vi "Calculate INL.vi"(8 "Error In":errorcluster, 10 "V Zero":dbl, 11 "ADC in":refnum<class "ADC.lvclass">) -> (0 "Error Out":errorcluster, 2 "INL":dbl[](array[numeric]), 3 "ADC out":refnum<class "ADC.lvclass">)   [LabVIEW 2023, in "ADC.lvclass"]
doc: "The VI calculates the INL values for the ADC."
uses:
  ADC.lvclass
  C:/Users/Ancy.Augustin/Downloads/Tasks (2)/Tasks/Tasks/SDLC - DNL and INL Testing/SDLC - DNL and INL Testing/INL and DNL Calculation/Classes/Mode/Mode.lvclass
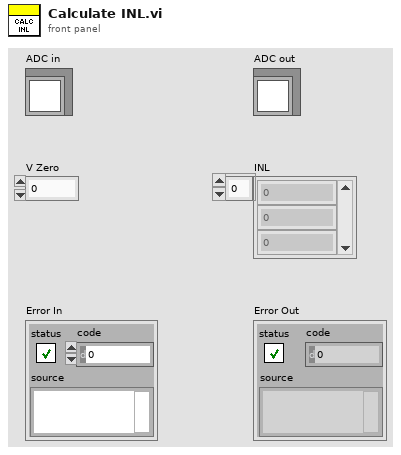
[diagram p1: front panel]
types:
  T1 = typedef "Transfer Function.ctl" = cluster{"Ideal voltage":dbl[], "Digital Code":dbl[]}
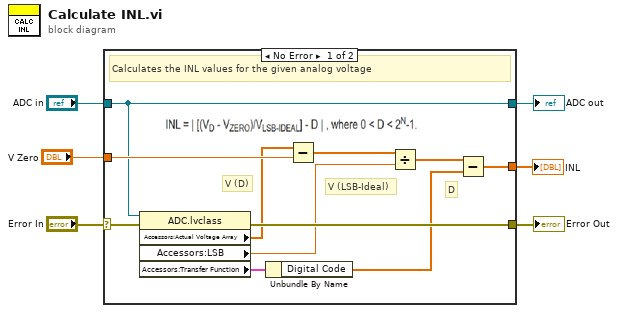
[diagram p0: block diagram]
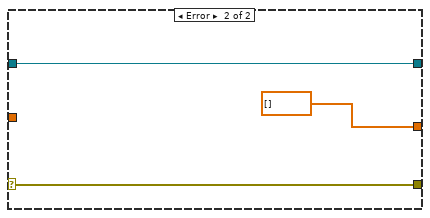
[diagram p2: hidden frame]
diagram:
  n1 = case shown="No Error" "Error In" {
    selector: "Error In" -> [w17 w20]
    tunnel: [w12 w20] -> w5
    tunnel: [w11 w19] -> w3
    tunnel: "ADC in" -> [w11 w19]
    tunnel: "V Zero" -> [w14 _]
    tunnel: [w13 dbl[] []] -> w1
    frame No Error {
      # "D"
      # "V (LSB-Ideal)"
      # "V (D)"
      # "Calculates the INL values for the given analog voltage"
      n2 = property class="ADC.lvclass"(reference=w11, error in=w17) -> (error out=w12:errorcluster, "Accessors:Actual Voltage Array"=w9:dbl[], "Accessors:LSB"=w8:dbl, "Accessors:Transfer Function"=w10:T1)  [unwired: 1 out]
      n3 = Unbundle By Name(w10) -> ("Digital Code"=w7:dbl[])
      n4 = Subtract(x=w9, y=w14) -> (x-y=w16:dbl[])
      n5 = Divide(x=w16, y=w8) -> (x/y=w15:dbl[])
      n6 = Subtract(x=w15, y=w7) -> (x-y=w13:dbl[])
    }
    frame Error {
    }
  }
  "Error Out" <- w5
  "ADC out" <- w3
  "INL" <- w1
